vi "Update Numeric Data.vi"(8 "error in (no error)":errorcluster, 10 "Numeric Data":u32, 11 "Status Updater in":refnum<class "Status Events.lvclass">) -> (0 "error out":errorcluster, 3 "Status Updater out":refnum<class "Status Events.lvclass">)   [LabVIEW 2014, in "Status Events.lvclass"]
uses:
  Status Events.lvclass
  Status Events.lvclass/Status Events.ctl
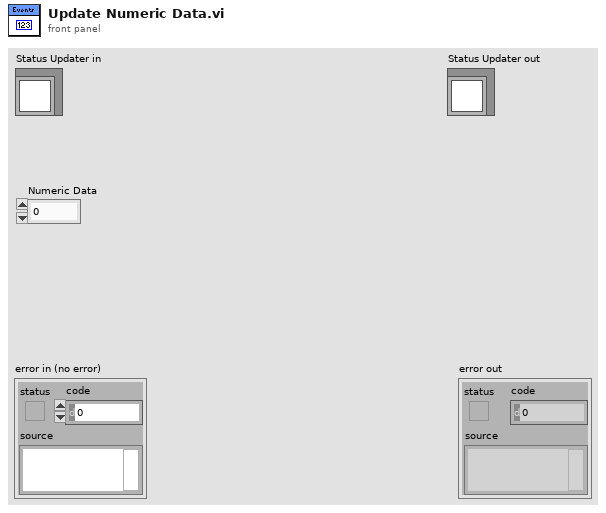
[diagram p1: front panel]
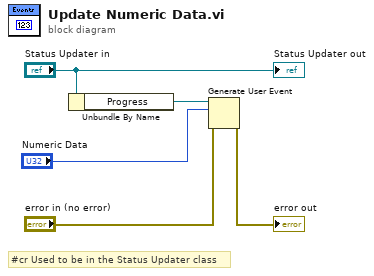
[diagram p0: block diagram]
diagram:
  # "#cr Used to be in the Status Updater class"
  n1 = Unbundle By Name("Status Updater in") -> ("Progress"=w5:refnum<user-event>)
  n2 = Generate User Event(user event=w5, event data cluster="Numeric Data", error in="error in (no error)") -> (error out=→"error out":errorcluster)  [unwired: 1 in, 1 out]
  "Status Updater out" <- "Status Updater in"
